vi "Engine.vi"() -> ()   [LabVIEW 2016]
panel:
  in  "Previous Button":bool
  # "ENGINE CONTROL"
  # "Next to you  is an element of the power part of the control system: \nMarching engine and two engines of angular stabilization.\nTo simulate the operation of the engine, a steam generator is used, a control element is presented for its use. \nYou must press the button for activate engine."
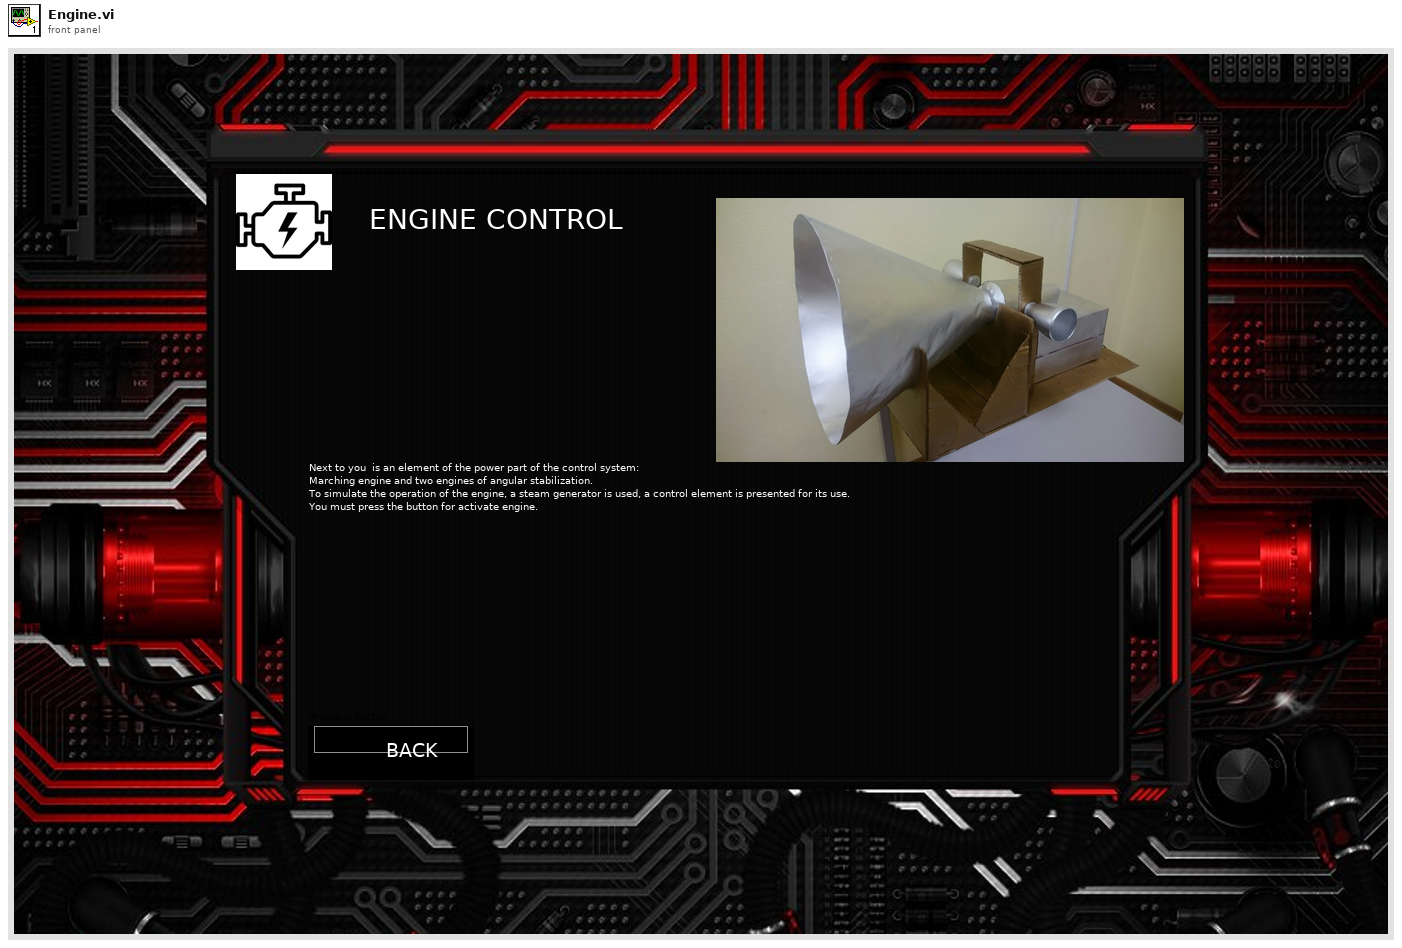
[diagram p1: front panel]
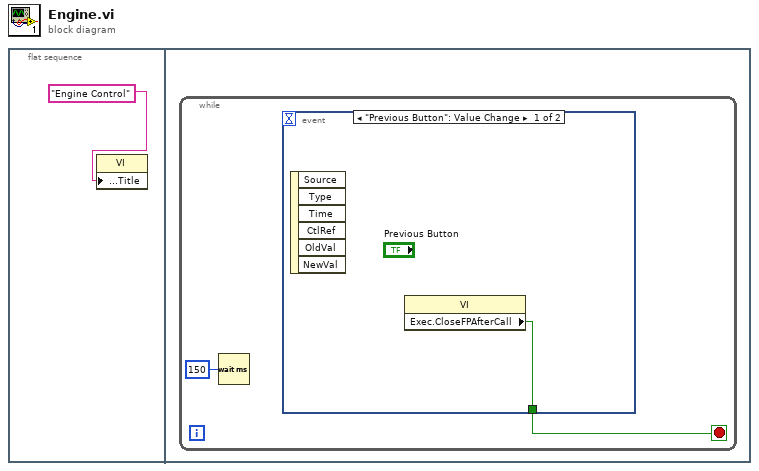
[diagram p0: block diagram]
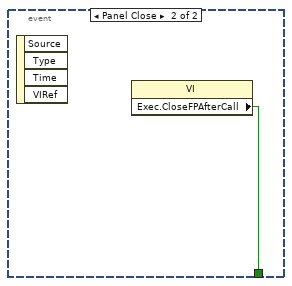
[diagram p2: hidden frame]
diagram:
  n1 = flat-sequence {
    frame #0 {
      n2 = property class="VI"("Front Panel.Title"="Engine Control" ("Front Panel Window:Title")) -> ()  [unwired: 2 in, 2 out]
    }
    frame #1 {
      n3 = while {
        stop <- w3 stop-if-true
        n4 = Wait (ms)(milliseconds to wait=u32 150) -> ()  [unwired: 1 out]
        n5 = event shown="[0] \"Previous Button\": Value Change" {
          selector: _ -> [_ _]
          dyn-events: _ -> [_ _]
          timeout: _ -> [_ _]
          tunnel: [w4 w5] -> w3
          event "Previous Button": Value Change {
            n6 = event-data() -> ()  [unwired: 1 in, 6 out]
            n7 = property class="VI"() -> ("Exec.CloseFPAfterCall"=w4:bool)  [unwired: 2 in, 2 out]
          }
          event Panel Close {
            n8 = event-data() -> ()  [unwired: 1 in, 4 out]
            n9 = property class="VI"() -> ("Exec.CloseFPAfterCall"=w5:bool)  [unwired: 2 in, 2 out]
          }
        }
      }
    }
  }
